vi "Calculate Mean Ignoring NaN.vi"(11 "Data in":sgl[](array[numeric])) -> (3 "Mean":sgl)   [LabVIEW 2015, in "Utility.lvlib"]
doc: "Calculates the mean of the numbers in <b>Data in</b> excluding any NaN."
uses:
  Utility.lvlib
  <vilib>/Analysis/baseanly.llb/Mean (DBL).vi
  <vilib>/Analysis/NI_AALBase.lvlib
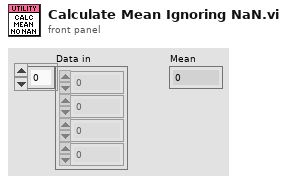
[diagram p1: front panel]
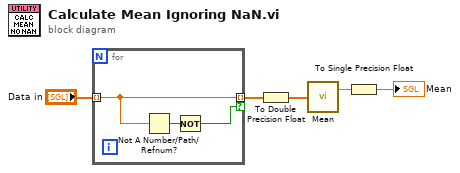
[diagram p0: block diagram]
diagram:
  n1 = for {
    tunnel: "Data in" -> [w8] mode=indexing
    tunnel: [w8] -> w2 mode=indexing if=w6
    n2 = Not A Number/Path/Refnum?(number/path/refnum=w8) -> (NaN/Path/Refnum?=w7:bool)
    n3 = Not(x=w7) -> (.not. x?=w6:bool)
  }
  n4 = To Double Precision Float(number=w2) -> (double precision float=w1:dbl[])
  n5 = call-poly <vilib>:"Mean.vi"("X"=w1) -> ("mean"=w4:dbl)  [unwired: 1 out]
  n6 = To Single Precision Float(number=w4) -> (single precision float=→"Mean":sgl)
